vi "f_p,L(y).vi"(9 "L":i32, 10 "p":i32, 11 "y":ext format="%#_4g") -> (3 "f_p,L(y)":ext format="%#_4g")   [LabVIEW 2019]
doc: "Recorded (saturated) signal per frame upon an incident signal with count rate mu detected by a SPAD with L accumulations per frame and recording in a counter with max value p\n\ny = e^-mu (0 <= y <= 1)\np = counter capacity (p >= 1)\nL = number of gate accumulation (L >= 1)\n\nFormula of 10/18/18"
uses:
  <vilib>/gmath/NI_Gmath.lvlib
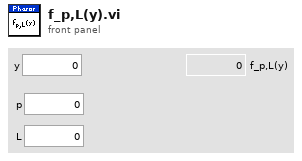
[diagram p1: front panel]
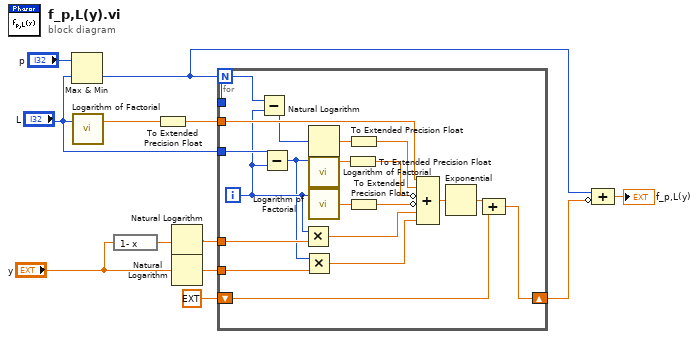
[diagram p0: block diagram]
diagram:
  n1 = Max & Min(x="p", y="L") -> (min(x,y)=w2:i32)  [unwired: 1 out]
  n2 = call <vilib>:"Logarithm of Factorial.vi"("n"="L") -> ("ln(n!)"=w12:dbl)  [unwired: 2 in]
  n3 = expression code="1- x"("y") -> (w11:ext)
  n4 = To Extended Precision Float(1:w12) -> (0:w1:ext)
  n5 = Natural Logarithm(1:w11) -> (0:w9:ext)
  n6 = Natural Logarithm(1:"y") -> (0:w8:ext)
  n7 = for {
    N: w2 -> [w26]
    tunnel: w1 -> [w32]
    tunnel: "L" -> [w29]
    tunnel: w9 -> [w31]
    tunnel: w8 -> [w30]
    shift-right: [w27] -> w5
    shift-left: ext 0.0 -> [w28]
    tunnel: w2 -> [_]
    i -> [w25]
    n8 = Subtract(x=w26, y=w25) -> (x-y=w23:i32)
    n9 = Subtract(x=w29, y=w25) -> (x-y=w24:i32)
    n10 = Multiply(x=w25, y=w31) -> (x*y=w19:ext)
    n11 = Multiply(x=w24, y=w30) -> (x*y=w18:ext)
    n12 = Natural Logarithm(1:w23) -> (0:w16:dbl)
    n13 = call <vilib>:"Logarithm of Factorial.vi"("n"=w24) -> ("ln(n!)"=w20:dbl)  [unwired: 2 in]
    n14 = call <vilib>:"Logarithm of Factorial.vi"("n"=w25) -> ("ln(n!)"=w21:dbl)  [unwired: 2 in]
    n15 = To Extended Precision Float(1:w20) -> (0:w14:ext)
    n16 = To Extended Precision Float(1:w16) -> (0:w15:ext)
    n17 = To Extended Precision Float(1:w21) -> (0:w13:ext)
    n18 = Compound Arithmetic op=ADD(w32, w15, invert w14, invert w13, w19, w18) -> (w17:ext)
    n19 = Exponential(1:w17) -> (0:w22:ext)
    n20 = Compound Arithmetic op=ADD(w22, w28) -> (w27:ext)
  }
  n21 = Compound Arithmetic op=ADD(w2, invert w5) -> (→"f_p,L(y)":ext)
